vi "mks670_get_uom.vi"() -> ()   [LabVIEW 2019]
panel:
  out "Unit":string
  out "Response":string
  out "Status":string
  in  "tpg361_visa 3":refnum<visa-resource-name>
  in  "err_in 2":errorcluster
  out "Overall Status":bool
  out "err_out":errorcluster
  out "tpg361_visa 2":refnum<visa-resource-name>
  in  "tpg361_b2r 2":u32
  in  "tpg361_delay 3":u32=500
  # "Status Notes:\n@ = Valid\n> = Parameter is unrecognized\n? = Invalid data field value\n= Inappropriate command"
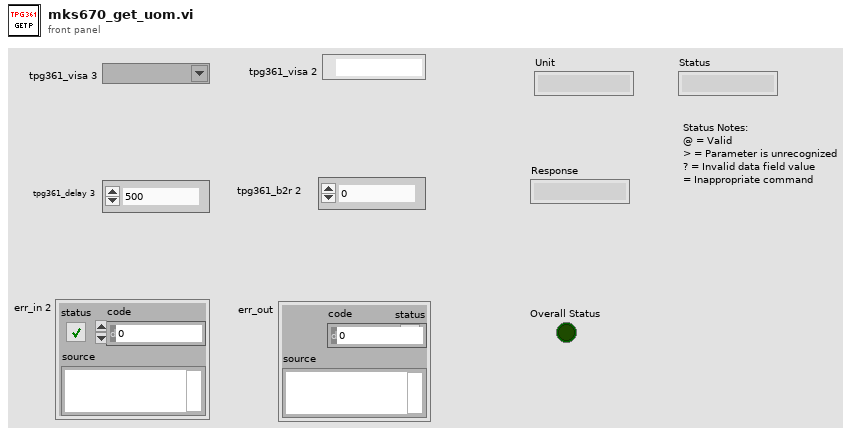
[diagram p1: front panel]
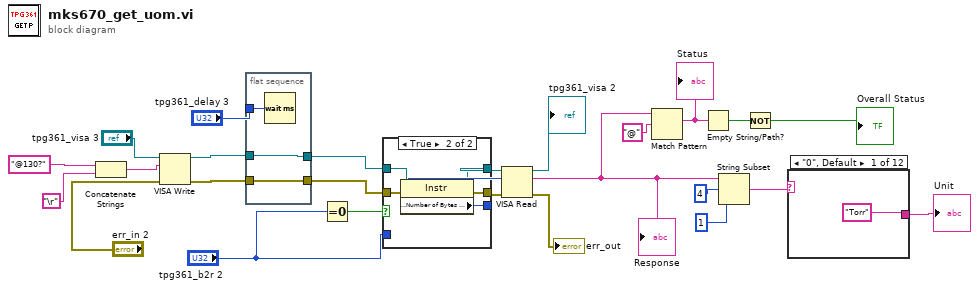
[diagram p0: block diagram]
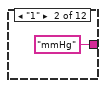
[diagram p2: hidden frame]
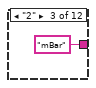
[diagram p3: hidden frame]
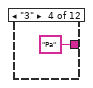
[diagram p4: hidden frame]
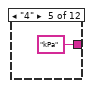
[diagram p5: hidden frame]
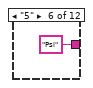
[diagram p6: hidden frame]
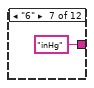
[diagram p7: hidden frame]
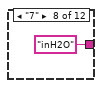
[diagram p8: hidden frame]
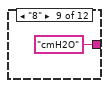
[diagram p9: hidden frame]
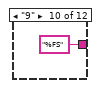
[diagram p10: hidden frame]
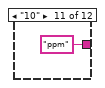
[diagram p11: hidden frame]
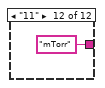
[diagram p12: hidden frame]
diagram:
  n1 = Concatenate Strings("@130?" ("write buffer"), "\r") -> (w7:string)
  n2 = VISA Write(VISA resource name="tpg361_visa 3", write buffer=w7, error in (no error)="err_in 2") -> (VISA resource name out=w20:refnum<visa-resource-name>, error out=w19:errorcluster)  [unwired: 1 out]
  n3 = flat-sequence {
    tunnel: [w28] -> w26
    tunnel: [w29] -> w25
    tunnel: w20 -> [w29]
    tunnel: w19 -> [w28]
    tunnel: "tpg361_delay 3" -> [w27]
    frame #0 {
      n4 = Wait (ms)(milliseconds to wait=w27) -> ()  [unwired: 1 out]
    }
  }
  n5 = Equal To 0?(x="tpg361_b2r 2") -> (x = 0?=w24:bool)
  n6 = case shown="True" w24 {
    tunnel: w26 -> [w31 w37]
    tunnel: w25 -> [w32 w36]
    tunnel: [w32 w35] -> w23
    tunnel: [w31 w34] -> w22
    tunnel: [w30 w33] -> w21
    tunnel: "tpg361_b2r 2" -> [w30 _]
    frame False {
    }
    frame True {
      n7 = property class="Instr"(reference=w36, error in=w37) -> (reference out=w35:refnum<visa-resource-name>, error out=w34:errorcluster, "Serial Settings:Number of Bytes at Serial Port"=w33:u32)
    }
  }
  n8 = VISA Read(VISA resource name=w23, byte count=w21, error in (no error)=w22) -> (VISA resource name out=→"tpg361_visa 2":refnum<visa-resource-name>, read buffer=w13:string, error out=→"err_out":errorcluster)  [unwired: 1 out]
  "Response" <- w13
  n9 = Match Pattern(string=w13, regular expression="@") -> (match substring=w11:string)  [unwired: 1 in, 3 out]
  "Status" <- w11
  n10 = Empty String/Path?(string/path=w11) -> (empty?=w10:bool)
  n11 = String Subset(string=w13, offset (0)=4, length (rest)=1 ("length (rest)")) -> (substring=w2:string)
  n12 = Not(x=w10) -> (.not. x?=→"Overall Status":bool)
  n13 = case shown="\"0\", Default" w2 {
    tunnel: ["Torr" "mmHg" "mBar" "Pa" "kPa" "Psi" "inHg" "inH2O" "cmH2O" "%FS" "ppm" "mTorr"] -> w1
    frame "0", Default {
    }
    frame "1" {
    }
    frame "2" {
    }
    frame "3" {
    }
    frame "4" {
    }
    frame "5" {
    }
    frame "6" {
    }
    frame "7" {
    }
    frame "8" {
    }
    frame "9" {
    }
    frame "10" {
    }
    frame "11" {
    }
  }
  "Unit" <- w1
